vi "Create Setting.vi"(8 "error in (no error)":errorcluster, 10 "Setting":T1, 11 "Path":path) -> (0 "error out":errorcluster)   [LabVIEW 2020, in "Logging.lvlib"]
uses:
  Logging.lvlib
  Define/Log Setting.ctl
  Define/Logger Setting.ctl
  Define/Log Option.ctl
  Define/Log Level.ctl
  <vilib>/Utility/xml.llb/Write to XML File(string).vi
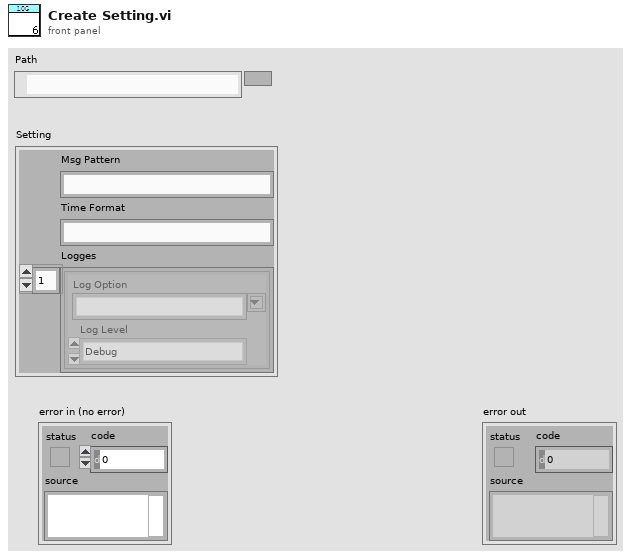
[diagram p1: front panel]
types:
  T1 = typedef "Logging.lvlib/Log Setting.ctl" = cluster{"Msg Pattern":string, "Time Format":string, "Logges":T2[]}
  T2 = typedef "Logging.lvlib/Logger Setting.ctl" = cluster{"Log Option":T3, "Log Level":T4}
  T3 = typedef "Logging.lvlib/Log Option.ctl" = string
  T4 = typedef "Logging.lvlib/Log Level.ctl" = enum16{"Debug", "Info", "Warn", "Error"}
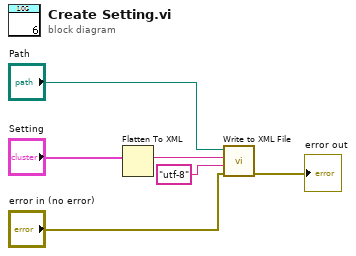
[diagram p0: block diagram]
diagram:
  n1 = Flatten To XML(6:"Setting") -> (2:w4:string)
  n2 = call-poly <vilib>:"Write to XML File.vi"("error in (no error)"="error in (no error)", "XML Encoding"="utf-8", "XML Input"=w4, "XML File Path"="Path") -> ("error out"=→"error out":errorcluster)  [unwired: 5 in, 2 out]
